vi "Random Number.vi"(1 "0 Base? (F)":bool, 2 "Min (0)":u32, 3 "Max":u32) -> (0 "Out":u32)   [LabVIEW 2018]
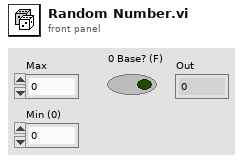
[diagram p1: front panel]
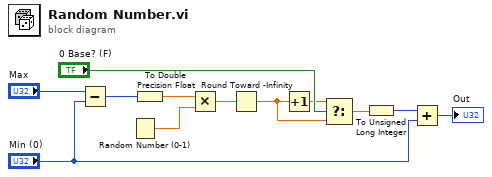
[diagram p0: block diagram]
diagram:
  n1 = Subtract(x="Max", y="Min (0)") -> (x-y=w7:u32)
  n2 = Random Number (0-1)() -> (number: 0 to 1=w12:dbl)
  n3 = To Double Precision Float(number=w7) -> (double precision float=w8:dbl)
  n4 = Multiply(x=w8, y=w12) -> (x*y=w10:dbl)
  n5 = Round Toward -Infinity(1:w10) -> (0:w3:dbl)
  n6 = Increment(x=w3) -> (x+1=w2:dbl)
  n7 = Select(t=w2, s="0 Base? (F)", f=w3) -> (s? t:f=w1:dbl)
  n8 = To Unsigned Long Integer(number=w1) -> (unsigned 32bit integer=w9:u32)
  n9 = Add(x=w9, y="Min (0)") -> (x+y=→"Out":u32)
